vi "GetWindowDisplayScale.vi"(8 "No Error":errorcluster, 11 "Window [SDL_Window *]":i64) -> (0 "error out":errorcluster, 3 "Display Scale":sgl)   [LabVIEW 2024, in "SDL3.lvlib" / "Video.lvlib"]
doc: "<B>Summary</B>\nGet the content display scale relative to a window's pixel size.\n\n<B>Remarks</B>\nThis is a combination of the window pixel density and the display content scale, and is the expected scale for displaying content in this window. For example, if a 3840x2160 window had a display scale of 2.0, the user expects the content to take twice as many pixels and be the same physical size as if it were being displayed in a 1920x1080 window with a display scale of 1.0.\n\nConceptually this value corresponds to the scale display setting, and is updated when that setting is changed, or the window moves to a display with a different scale setting.\n\nNote: This function may fail on systems where the window has not yet been decorated by the display server (for example, immediately after calling SDL_CreateWindow). It is recommended that you wait at least until the window has been presented and composited, so that the window system has a chance to decorate the window and provide the border dimensions to SDL.\n\nThis function also returns false if getting the information is not supported."
uses:
  Video.lvlib
  Error/Error.lvlib
  Lib/SDL3-32.dll
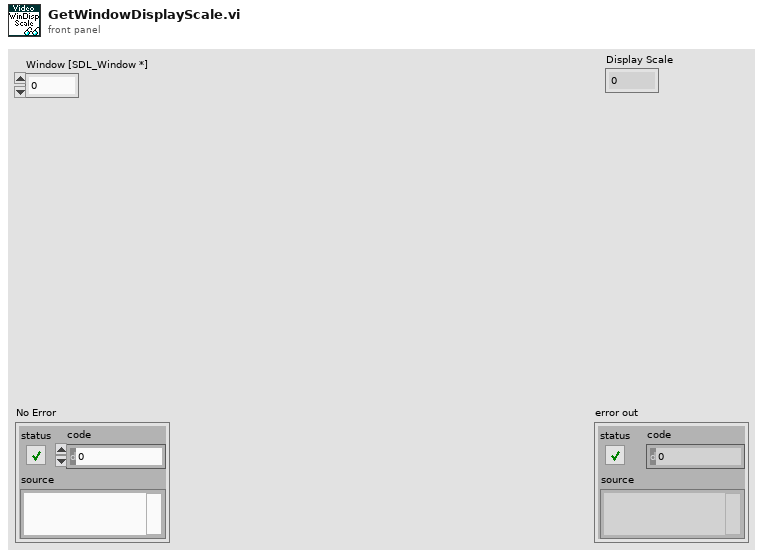
[diagram p1: front panel]
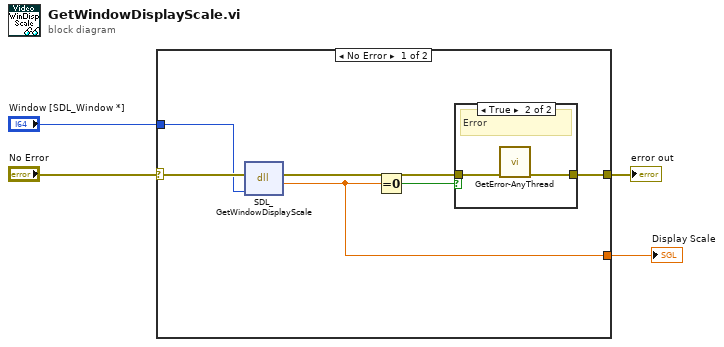
[diagram p0: block diagram]
diagram:
  n1 = case shown="No Error" "No Error" {
    selector: "No Error" -> [w10 w14]
    tunnel: [w7 w14] -> w3
    tunnel: "Window [SDL_Window *]" -> [w9 _]
    tunnel: [w6 _] -> w1
    frame No Error {
      n2 = dll-call lib="C:/Users/Thomas/Documents/Projects/LV-SDL3/Lib/SDL3-*.*" fn="SDL_GetWindowDisplayScale"(error in=w10, "window"=w9) -> (error out=w8:errorcluster, "return type"=w6:sgl)  [unwired: 3 in, 1 out]
      n3 = Equal To 0?(x=w6) -> (x = 0?=w5:bool)
      n4 = case shown="True" w5 {
        tunnel: w8 -> [w11 w13]
        tunnel: [w11 w12] -> w7
        frame False {
          # "Ok"
        }
        frame True {
          # "Error"
          n5 = call "GetError-AnyThread.vi"("No Error"=w13) -> ("error out"=w12:errorcluster)  [unwired: 10 in]
        }
      }
    }
    frame Error {
    }
  }
  "error out" <- w3
  "Display Scale" <- w1
